vi "Parse VIs.vi"(8 "Error In":errorcluster, 10 "All VIs":path[](array[path]), 11 "Doc Config":T1) -> (0 "Error Out":errorcluster, 2 "VIs":T2[](array[typedef]), 3 "Doc Config":T1)   [LabVIEW 2011, in "LMH-Toolbox.lvlib" / "LMH-Documentation.lvlib"]
uses:
  LMH-Documentation.lvlib
  Type Defs/VI.ctl
  Type Defs/Doc Config.ctl
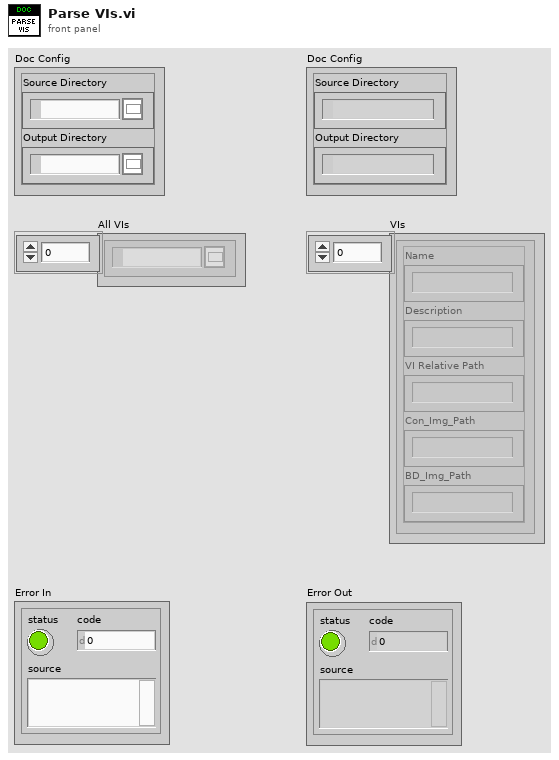
[diagram p1: front panel]
types:
  T1 = typedef "LMH-Toolbox.lvlib/LMH-Documentation.lvlib/Doc Config.ctl" = cluster{"Source Directory":path, "Output Directory":path}
  T2 = typedef "LMH-Toolbox.lvlib/LMH-Documentation.lvlib/VI.ctl" = cluster{"Name":string, "Description":string, "VI Relative Path":string, "Con_Img_Path":string, "BD_Img_Path":string}
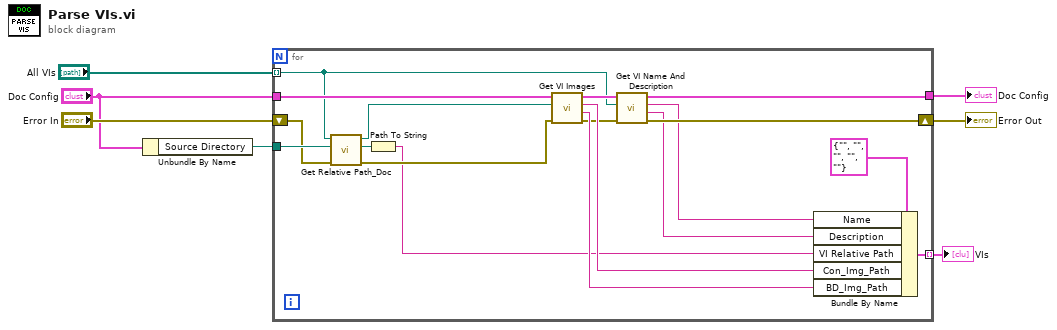
[diagram p0: block diagram]
diagram:
  n1 = Unbundle By Name("Doc Config") -> ("Source Directory"=w1:path)
  n2 = for {
    tunnel: "Doc Config" -> [w15]
    tunnel: "All VIs" -> [w11] mode=indexing
    shift-right: [w20] -> w4
    shift-left: "Error In" -> [w13]
    tunnel: [w22] -> w7 mode=indexing
    tunnel: [w16] -> w3
    tunnel: w1 -> [w14]
    n3 = call "Get Relative Path_Doc.vi"("Error In"=w13, "Relative Path Root"=w14, "File / Folder"=w11) -> ("Error Out"=w12:errorcluster, "Relative Path"=w9:path, "Duplicate File / Folder"=w10:path)  [unwired: 6 in]
    n4 = Path To String(path=w9) -> (string=w8:string)
    n5 = call "Get VI Images.vi"("Error In"=w12, "VI Path"=w10, "Doc Config"=w15) -> ("Error Out"=w21:errorcluster, "BD_Img_Path"=w23:string, "Con_Img_Path"=w24:string, "Doc Config"=w19:T1)  [unwired: 5 in]
    n6 = call "Get VI Name And Description.vi"("Error In"=w21, "VI Path"=w11, "Doc Config"=w19) -> ("Error Out"=w20:errorcluster, "VI Description"=w17:string, "VI Name"=w18:string, "Doc Config"=w16:T1)  [unwired: 5 in]
    n7 = Bundle By Name(cluster=T2 {"Name"="", "Description"="", "VI Relative Path"="", "Con_Img_Path"="", "BD_Img_Path"=""} ("VI"), "Name"=w18, "Description"=w17, "VI Relative Path"=w8, "Con_Img_Path"=w24, "BD_Img_Path"=w23) -> (w22:T2)
  }
  "VIs" <- w7
  "Error Out" <- w4
  "Doc Config" <- w3
